vi "PWM DC Cmd.vi"(8 "error in (no error)":errorcluster, 9 "Board Selector":T3, 10 "Array in":T2(array[cluster]), 11 "VISA Refnum in":refnum<visa-resource-name>) -> (0 "error out":errorcluster, 2 "Array out":dbl[](array[numeric]), 3 "VISA Refnum out":refnum<visa-resource-name>)   [LabVIEW 2022 SP3]
uses:
  Serial Board Com/Board Select.ctl
  Serial Board Com/ADCSelector BB.ctl
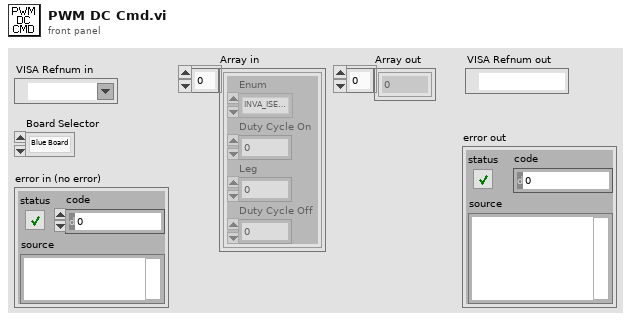
[diagram p1: front panel]
types:
  T1 = typedef "ADCSelector BB.ctl" = enum16{"INVA_ISENSE_U", "INVA_ISENSE_V", "INVA_ISENSE_W", "INVA_UDC", "INVA_TEMP", "HB_TEMP", "AUXB_TEMP", "VLINE_AB", "VLINE_BC", "VLINE_CA", "VSENSE_POS_24V", "VSENSE_POS_5V", "VSENSE_NEG_15V", "INVB_ISENSE_U", "INV_B_ISENSEV", "INVB_ISENSE_W", "INVB_UDC", "INVB_TEMP", "AUXA_TEMP", "AUXC_TEMP", "VOUT_AB", "VOUT_BC", "VOUT_CA", "VSENSE_POS_15V", "VSENSE_POS_3P3V", "TEST_POINT"}
  T2 = cluster{"Enum":T1, "Duty Cycle On":i32, "Leg":i32, "Duty Cycle Off":i32}[]
  T3 = typedef "Board Select.ctl" = enum16{"Blue Board", "Green Board"}
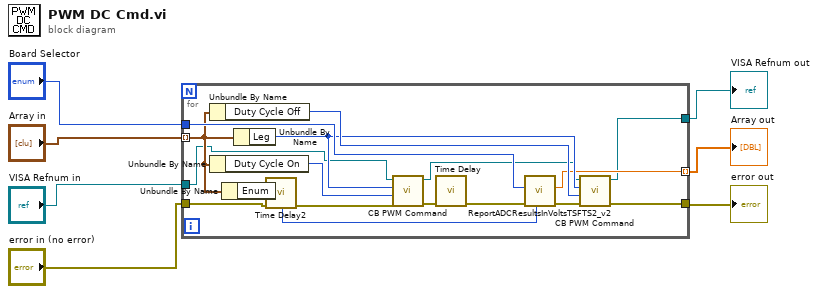
[diagram p0: block diagram]
diagram:
  n1 = for {
    tunnel: "Array in" -> [w17] mode=indexing
    tunnel: "Board Selector" -> [w22]
    tunnel: [w14] -> w5 mode=indexing
    tunnel: [w13] -> w2
    tunnel: "error in (no error)" -> [w12]
    tunnel: "VISA Refnum in" -> [w10]
    tunnel: [w8] -> w1
    n2 = Unbundle By Name(w17) -> ("Duty Cycle Off"=w16:i32)
    n3 = Unbundle By Name(w17) -> ("Duty Cycle On"=w21:i32)
    n4 = Unbundle By Name(w17) -> ("Enum"=w23:T1)
    n5 = Unbundle By Name(w17) -> ("Leg"=w15:i32)
    n6 = call "Time Delay2"("error in (no error)"=w12) -> ("error out"=w11:errorcluster)  [unwired: 10 in]
    n7 = call "CB PWM Command.vi"("error in (no error)"=w11, "Duty Cycle"=w21, "Leg"=w15, "VISA Refnum in"=w10) -> ("error out"=w20:errorcluster, "VISA Refnum out"=w9:refnum<visa-resource-name>)  [unwired: 5 in, 1 out]
    n8 = call "Time Delay"("error in (no error)"=w20) -> ("error out"=w19:errorcluster)  [unwired: 10 in]
    n9 = call "ReportADCResultsInVoltsTSFTS2_v2.vi"("Blue Board Enum"=w23, "error in (no error)"=w19, "Board Selector"=w22) -> ("error out"=w18:errorcluster, "Result"=w14:dbl)  [unwired: 5 in, 2 out]
    n10 = call "CB PWM Command.vi"("error in (no error)"=w18, "Duty Cycle"=w16, "Leg"=w15, "VISA Refnum in"=w9) -> ("error out"=w13:errorcluster, "VISA Refnum out"=w8:refnum<visa-resource-name>)  [unwired: 5 in, 1 out]
  }
  "Array out" <- w5
  "error out" <- w2
  "VISA Refnum out" <- w1
